vi "factorial (SubVI).vi"(11 "Num":i32) -> (3 "Numeric":u64)   [LabVIEW 2023]
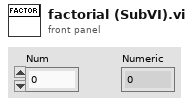
[diagram p1: front panel]
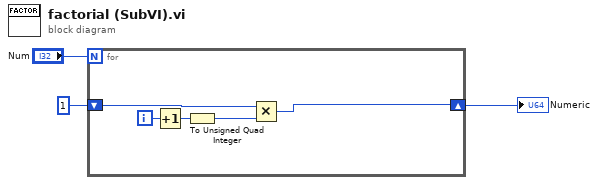
[diagram p0: block diagram]
diagram:
  n1 = for {
    N: "Num" -> [_]
    shift-right: [w5] -> w2
    shift-left: u64 1 -> [w7]
    i -> [w8]
    n2 = Increment(x=w8) -> (x+1=w6:i32)
    n3 = To Unsigned Quad Integer(1:w6) -> (0:w4:u64)
    n4 = Multiply(x=w7, y=w4) -> (x*y=w5:u64)
  }
  "Numeric" <- w2
